vi "iWorx Event Marker SubVI.vi"(7 "Reset count (f)":bool, 11 "waveform in":waveform(dbl)) -> (0 "Button Press Duration":dbl, 1 "Two Edge Separation (rising)":dbl, 2 "Button State":bool, 3 "0-1 Waveform out":waveform(dbl), 4 "Falling Edge Times":timestamp[](array[timestamp]), 5 "Button Count":u32, 6 "Rising Edge Times":timestamp[](array[timestamp]))   [LabVIEW 2012]
doc: "This subVI is designed to work with the iWorx Event Marker. It takes in a waveform from the sensor and records timestamps for each rising and falling edge."
uses:
  <vilib>/ptbypt/NI_PtbyPt.lvlib
panel:
  out "rounded":dbl=10.0
  out "raw":dbl=10.0
  in  "# of Timestamps to store":i32=10
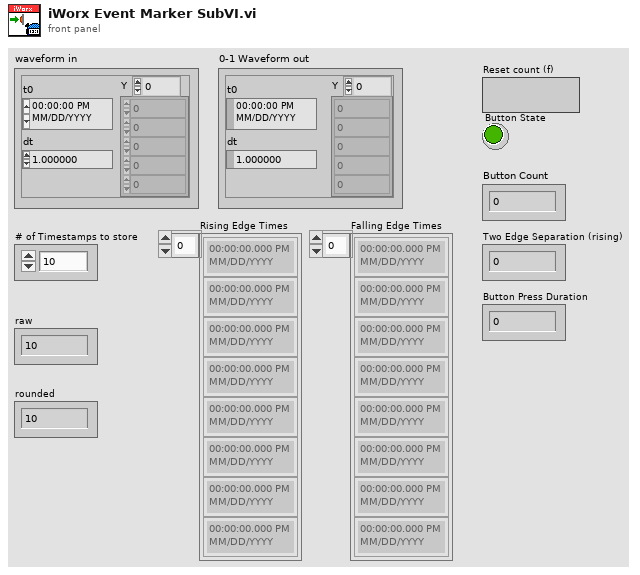
[diagram p1: front panel]
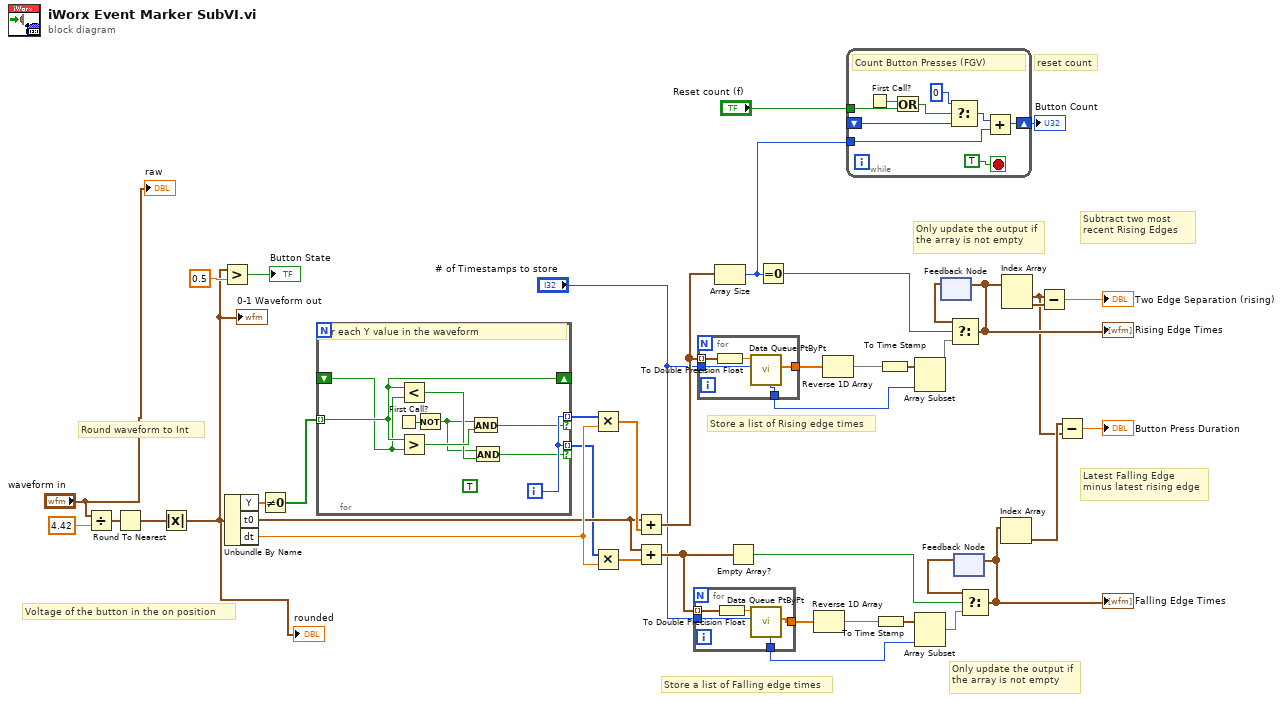
[diagram p0: block diagram]
diagram:
  # "reset count"
  # "Round waveform to Int"
  # "Latest Falling Edge minus latest rising edge"
  # "Subtract two most recent Rising Edges"
  # "Only update the output if the array is not empty"
  # "Only update the output if the array is not empty"
  # "Store a list of Rising edge times"
  # "Store a list of Falling edge times"
  # "Voltage of the button in the on position"
  n1 = Divide(x="waveform in", y=4.42) -> (x/y=w18:waveform(dbl))
  n2 = Round To Nearest(number=w18) -> (nearest integer value=w2:waveform(dbl))
  n3 = Absolute Value(x=w2) -> (abs(x)=w1:waveform(dbl))
  "0-1 Waveform out" <- w1
  "rounded" <- w1
  n4 = Greater?(x=w1, y=0.5 ("x")) -> (0:→"Button State":bool)
  n5 = Unbundle By Name(w1) -> ("Y"=w40:dbl[], "t0"=w34:timestamp, "dt"=w37:dbl)
  n6 = Not Equal To 0?(x=w40) -> (x != 0?=w39:bool[])
  n7 = for {
    tunnel: [w51] -> w33 mode=indexing if=w50
    tunnel: [w51] -> w38 mode=indexing if=w49
    tunnel: w39 -> [w48] mode=indexing
    shift-right: [w48] -> _
    shift-left: _ -> [w47]
    i -> [w51]
    (unwired) TRUE
    # "For each Y value in the waveform"
    n8 = First Call?() -> (First Call?: T/F=w43:bool)
    n9 = Less?(x=w48, y=w47) -> (x < y?=w45:bool)
    n10 = Greater?(x=w48, y=w47) -> (0:w46:bool)
    n11 = Not(x=w43) -> (.not. x?=w44:bool)
    n12 = And(x=w44, y=w46) -> (x .and. y?=w49:bool)
    n13 = And(x=w44, y=w45) -> (x .and. y?=w50:bool)
  }
  n14 = Multiply(x=w38, y=w37) -> (x*y=w36:dbl[])
  n15 = Multiply(x=w33, y=w37) -> (x*y=w35:dbl[])
  n16 = Add(x=w34, y=w36) -> (x+y=w29:timestamp[])
  n17 = Add(x=w34, y=w35) -> (x+y=w11:timestamp[])
  n18 = for {
    tunnel: w11 -> [w55] mode=indexing
    tunnel: "# of Timestamps to store" -> [w56]
    tunnel: [w53] -> w6
    tunnel: [w52] -> w13
    n19 = To Double Precision Float(number=w55) -> (double precision float=w54:dbl)
    n20 = call <vilib>:"Data Queue PtByPt.vi"("sample length"=w56, "input data point"=w54) -> ("Current Queue"=w53:dbl[], "current length"=w52:i32)  [unwired: 5 in, 3 out]
  }
  n21 = for {
    tunnel: w29 -> [w60] mode=indexing
    tunnel: "# of Timestamps to store" -> [w61]
    tunnel: [w58] -> w8
    tunnel: [w57] -> w15
    n22 = To Double Precision Float(number=w60) -> (double precision float=w59:dbl)
    n23 = call <vilib>:"Data Queue PtByPt.vi"("sample length"=w61, "input data point"=w59) -> ("Current Queue"=w58:dbl[], "current length"=w57:i32)  [unwired: 5 in, 3 out]
  }
  n24 = Array Size(array=w29) -> (size(s)=w28:i32)
  n25 = Empty Array?(array=w11) -> (empty?=w19:bool)
  n26 = Equal To 0?(x=w28) -> (x = 0?=w24:bool)
  n27 = Reverse 1D Array(array=w6) -> (reversed array=w5:dbl[])
  n28 = Reverse 1D Array(array=w8) -> (reversed array=w7:dbl[])
  n29 = while {
    shift-right: [w62] -> w27
    shift-left: _ -> [w64]
    tunnel: w28 -> [w66]
    tunnel: "Reset count (f)" -> [w65]
    stop <- TRUE stop-if-true
    # "Count Button Presses (FGV)"
    n30 = First Call?() -> (First Call?: T/F=w69:bool)
    n31 = Or(x=w69, y=w65) -> (x .or. y?=w67:bool)
    n32 = Select(t=u32 0, s=w67, f=w64) -> (s? t:f=w63:u32)
    n33 = Add(x=w63, y=w66) -> (x+y=w62:u32)
  }
  "Button Count" <- w27
  n34 = To Time Stamp(1:w5) -> (0:w12:timestamp[])
  n35 = To Time Stamp(1:w7) -> (0:w16:timestamp[])
  n36 = Array Subset(array=w16, length=w15) -> (w14:timestamp[])  [unwired: 1 in]
  n37 = Array Subset(array=w12, length=w13) -> (w9:timestamp[])  [unwired: 1 in]
  n38 = feedback #1() -> (w32:timestamp[])  [unwired: 1 in]
  n39 = Select(t=w32, s=w24, f=w14) -> (s? t:f=w31:timestamp[])
  "Rising Edge Times" <- w31
  n40 = feedback-in #1(w31) -> ()
  n41 = feedback #2() -> (w30:timestamp[])  [unwired: 1 in]
  n42 = Select(t=w30, s=w19, f=w9) -> (s? t:f=w23:timestamp[])
  "Falling Edge Times" <- w23
  n43 = feedback-in #2(w23) -> ()
  n44 = Index Array(array=w23) -> (element=w21:timestamp)  [unwired: 1 in]
  n45 = Index Array(array=w31) -> (element #1=w20:timestamp, element #2=w41:timestamp)  [unwired: 2 in]
  n46 = Subtract(x=w20, y=w41) -> (x-y=→"Two Edge Separation (rising)":dbl)
  n47 = Subtract(x=w21, y=w20) -> (x-y=→"Button Press Duration":dbl)
  "raw" <- "waveform in"
